vi "DataProcess_CalcTorque.vi"(8 "error in (no error)":errorcluster, 11 "Path":path) -> (0 "error out":errorcluster, 1 "AverageTorque":T1, 2 "Torques":T3, 3 "Torque Errors":T2, 5 "ExtraWeight(kg)":cluster{"Thigh":dbl, "Shank":dbl}, 7 "match substring":string)   [LabVIEW 2015]
uses:
  CAlex2-Data/CAlex2_Data.lvclass
  <vilib>/Analysis/5stat.llb/RMS (DBL).vi
  <vilib>/Analysis/NI_AALPro.lvlib
panel:
  out "Planned Torque 4":dbl[][](graph)
  out "Planned Torque 3":dbl[][](graph)
  out "PID Error":dbl[](array[numeric])
  out "Planning Error":dbl[](array[numeric])
  out "All Error":dbl[](array[numeric])
  out "Planed Torque":dbl[][](graph)
  out "Desired Torque":dbl[][](graph)
  out "Acutal Torque":dbl[][](graph)
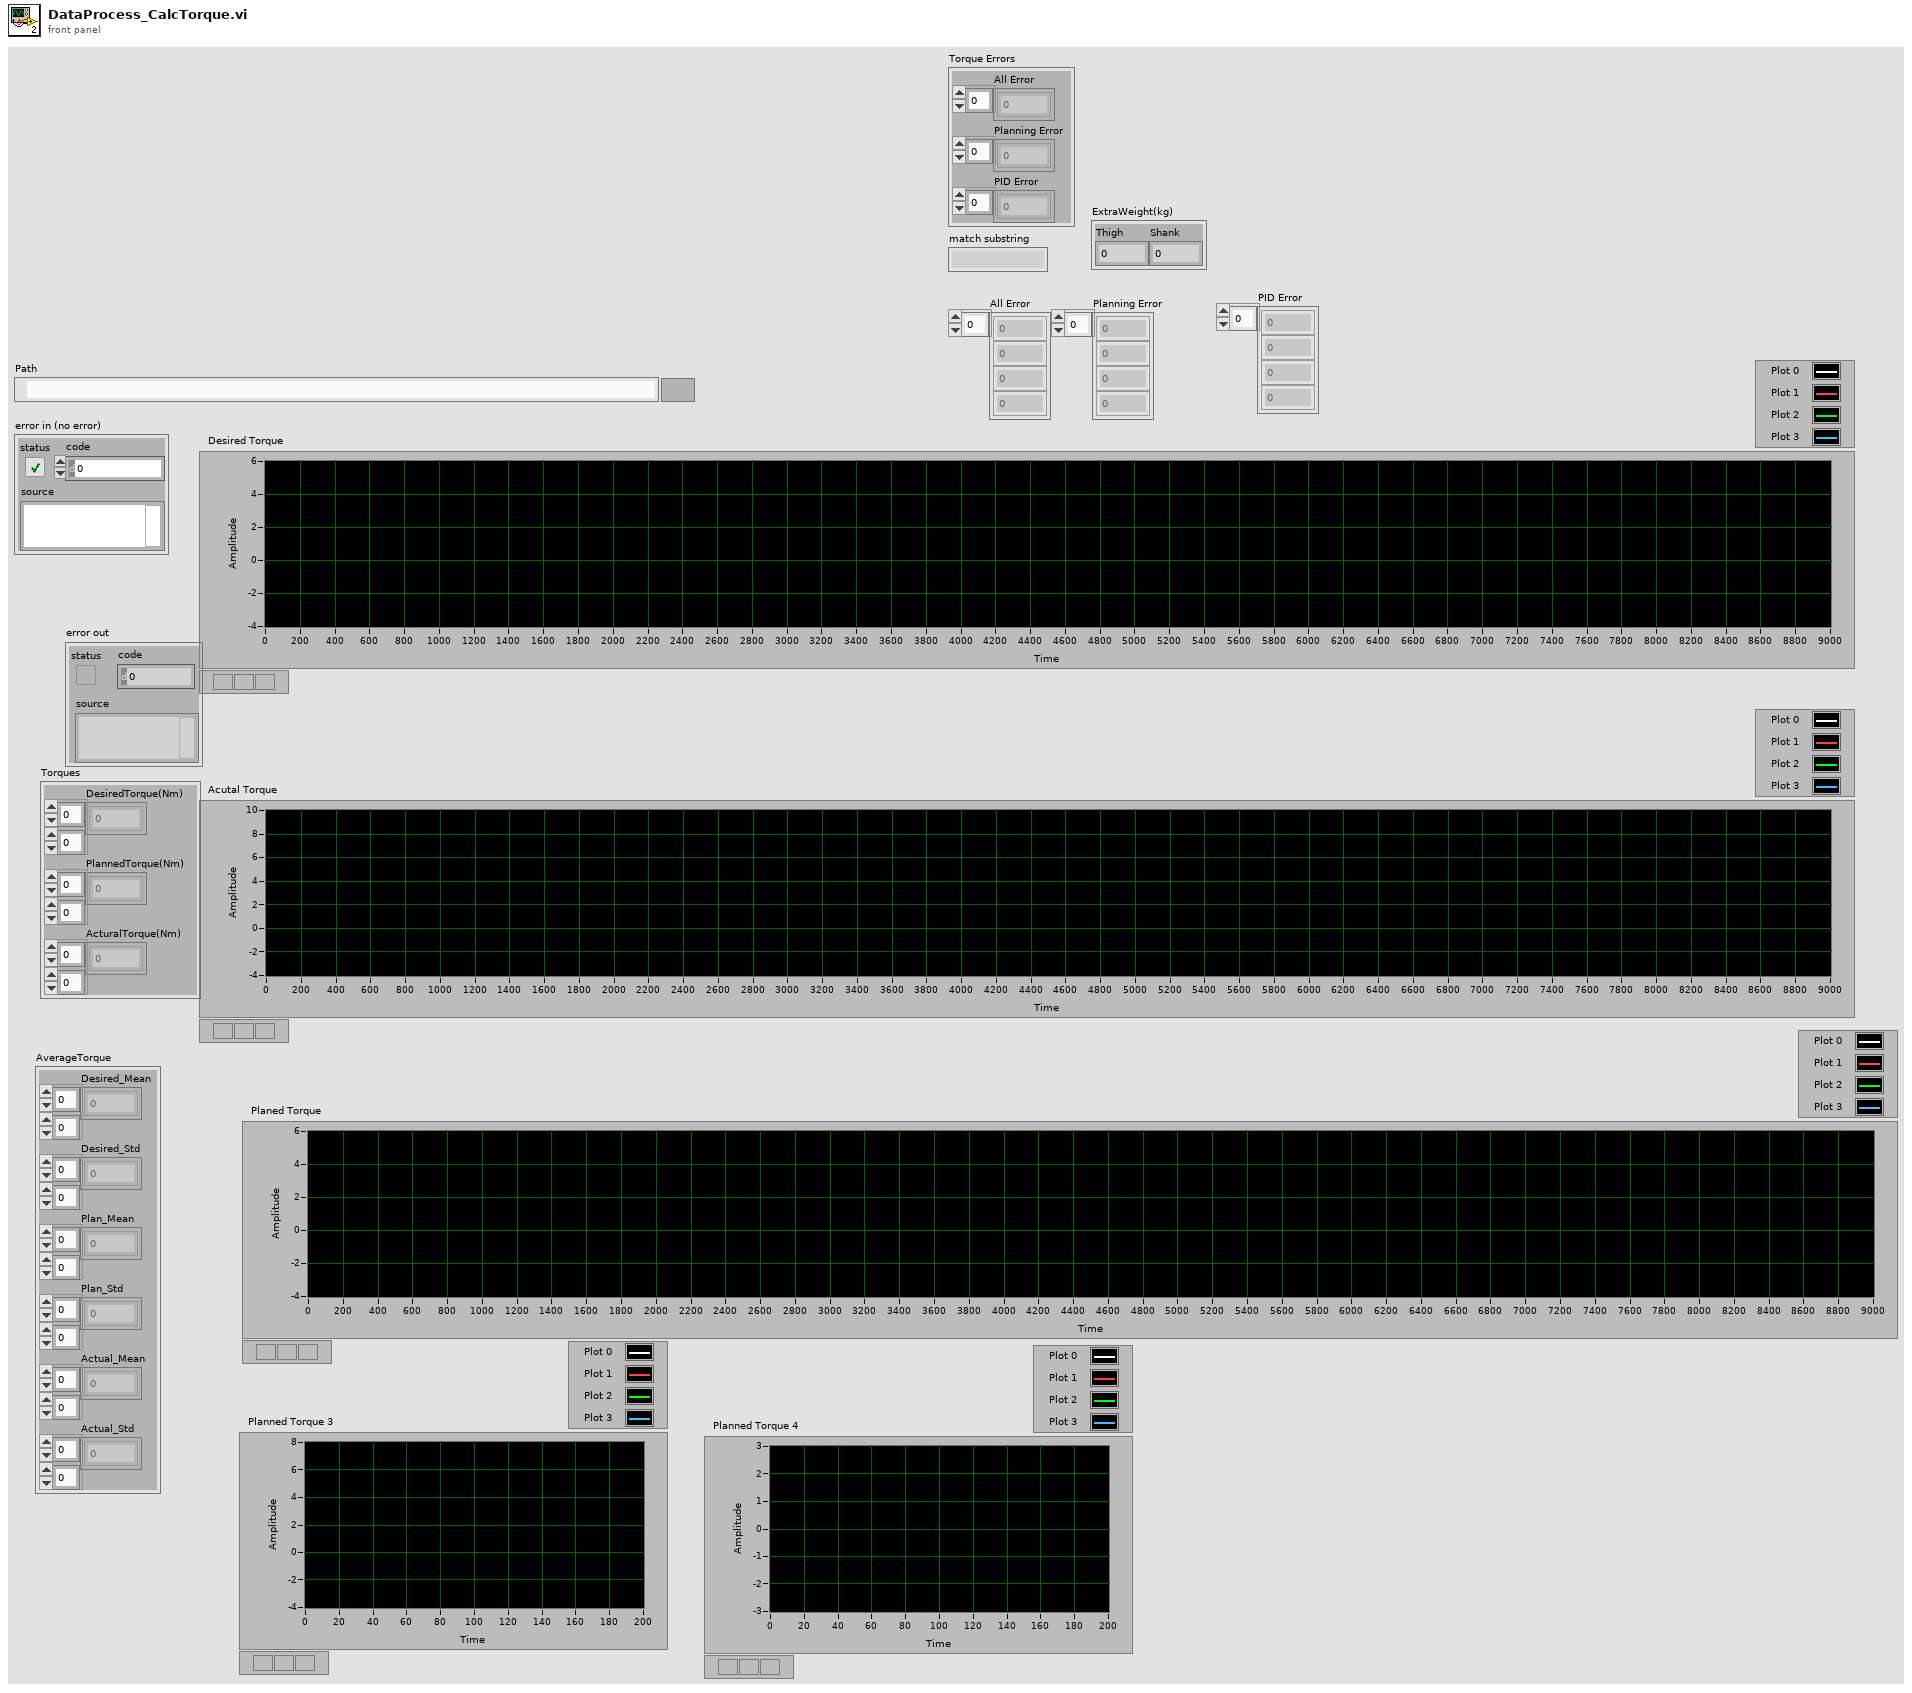
[diagram p1: front panel]
types:
  T1 = cluster{"Desired_Mean":dbl[][], "Desired_Std":dbl[][], "Plan_Mean":dbl[][], "Plan_Std":dbl[][], "Actual_Mean":dbl[][], "Actual_Std":dbl[][]}
  T2 = cluster{"All Error":dbl[], "Planning Error":dbl[], "PID Error":dbl[]}
  T3 = cluster{"DesiredTorque(Nm)":dbl[][], "PlannedTorque(Nm)":dbl[][], "ActuralTorque(Nm)":dbl[][]}
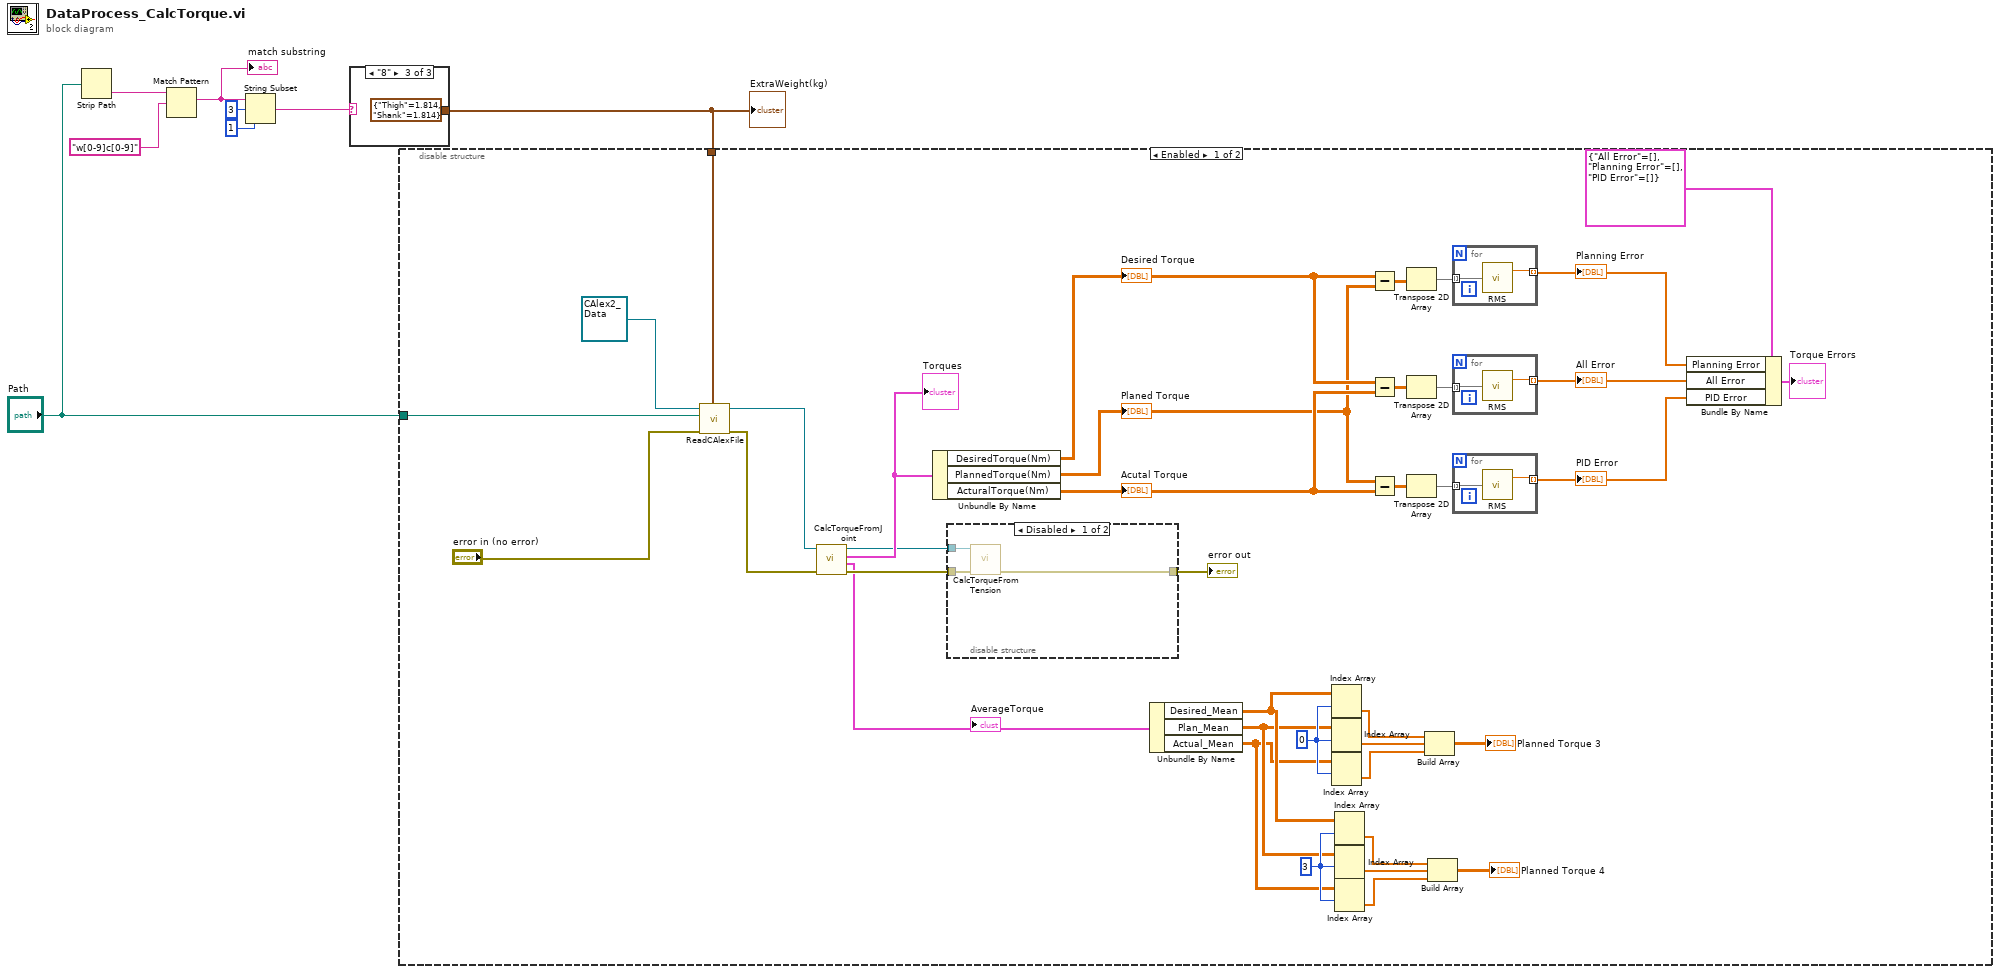
[diagram p0: block diagram]
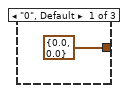
[diagram p4: hidden frame]
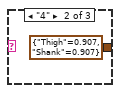
[diagram p5: hidden frame]
diagram:
  n1 = Strip Path(path="Path") -> (name=w7:string)  [unwired: 1 out]
  n2 = Match Pattern(string=w7, regular expression="w[0-9]c[0-9]") -> (match substring=w5:string)  [unwired: 1 in, 3 out]
  "match substring" <- w5
  n3 = String Subset(string=w5, offset (0)=3, length (rest)=1 ("length (rest)")) -> (substring=w2:string)
  n4 = case shown="\"8\"" w2 {
    tunnel: [cluster{"Thigh":dbl, "Shank":dbl} {"Thigh"=0.0, "Shank"=0.0} ("ExtraWeight(kg)") cluster{"Thigh":dbl, "Shank":dbl} {"Thigh"=0.907, "Shank"=0.907} ("ExtraWeight(kg)") cluster{"Thigh":dbl, "Shank":dbl} {"Thigh"=1.814, "Shank"=1.814} ("ExtraWeight(kg)")] -> w1
    frame "0", Default {
    }
    frame "4" {
    }
    frame "8" {
    }
  }
  "ExtraWeight(kg)" <- w1
  n5 = disable-structure shown="Enabled" {
    disable-tunnel: "Path" -> [w33 _]
    disable-tunnel: w1 -> [w31 _]
    frame Enabled {
      w19 = 3 ("index (row)")
      w20 = 0 ("index (row)")
      n6 = call "ReadCAlexFile.vi"("ExtraWeight(kg)"=w31, "error in (no error)"="error in (no error)", "ExpData File Path"=w33, "CAlexData2"=refnum<class "CAlex2_Data.lvclass"> refnum) -> ("error out"=w46:errorcluster, "CAlexData 2"=w47:refnum<class "CAlex2_Data.lvclass">)  [unwired: 6 in]
      n7 = call "CalcTorqueFromJoint.vi"("error in (no error)"=w46, "CAlexData2 in"=w47) -> ("error out"=w43:errorcluster, "AverageTorque"=w25:T1, "Torques"=w45:T3, "CarexMData out"=w44:refnum<class "CAlex2_Data.lvclass">)  [unwired: 5 in, 1 out]
      "Torques" <- w45
      "AverageTorque" <- w25
      n8 = Unbundle By Name(w45) -> ("DesiredTorque(Nm)"=w42:dbl[][], "PlannedTorque(Nm)"=w38:dbl[][], "ActuralTorque(Nm)"=w39:dbl[][])
      "Acutal Torque" <- w39
      "Desired Torque" <- w42
      "Planed Torque" <- w38
      n9 = disable-structure shown="Disabled" {
        disable-tunnel: w44 -> [w54 _]
        disable-tunnel: w43 -> [w53 w55]
        disable-tunnel: [w50 w55] -> w32
        frame Disabled {
          n10 = call "CalcTorqueFromTension.vi"("error in (no error)"=w53, "CAlexData2 in"=w54) -> ("error out"=w50:errorcluster, "Joint Torque Actual"=w51:dbl[][], "Joint Torque Desired"=w52:dbl[][])  [unwired: 4 in, 3 out]
        }
        frame Enabled {
        }
      }
      "error out" <- w32
      n11 = Unbundle By Name(w25) -> ("Desired_Mean"=w14:dbl[][], "Plan_Mean"=w13:dbl[][], "Actual_Mean"=w12:dbl[][])
      n12 = Index Array(array=w14, index (row)=w20) -> (element=w22:dbl[])  [unwired: 1 in]
      n13 = Index Array(array=w13, index (row)=w20) -> (element=w23:dbl[])  [unwired: 1 in]
      n14 = Index Array(array=w12, index (row)=w20) -> (element=w24:dbl[])  [unwired: 1 in]
      n15 = Index Array(array=w14, index (row)=w19) -> (element=w17:dbl[])  [unwired: 1 in]
      n16 = Index Array(array=w13, index (row)=w19) -> (element=w16:dbl[])  [unwired: 1 in]
      n17 = Index Array(array=w12, index (row)=w19) -> (element=w15:dbl[])  [unwired: 1 in]
      n18 = Subtract(x=w42, y=w38) -> (x-y=w41:dbl[][])
      n19 = Subtract(x=w42, y=w39) -> (x-y=w36:dbl[][])
      n20 = Subtract(x=w38, y=w39) -> (x-y=w34:dbl[][])
      n21 = Transpose 2D Array(2D array=w41) -> (transposed array=w40:dbl[][])
      n22 = Transpose 2D Array(2D array=w36) -> (transposed array=w37:dbl[][])
      n23 = Transpose 2D Array(2D array=w34) -> (transposed array=w35:dbl[][])
      n24 = Build Array(w22, w23, w24) -> (→"Planned Torque 3":dbl[][])
      n25 = Build Array(w17, w16, w15) -> (→"Planned Torque 4":dbl[][])
      n26 = for {
        tunnel: w40 -> [w61] mode=indexing
        tunnel: [w60] -> w30 mode=indexing
        n27 = call-poly <vilib>:"RMS.vi"("X"=w61) -> ("rms value"=w60:dbl)  [unwired: 1 out]
      }
      "Planning Error" <- w30
      n28 = for {
        tunnel: w37 -> [w59] mode=indexing
        tunnel: [w58] -> w29 mode=indexing
        n29 = call-poly <vilib>:"RMS.vi"("X"=w59) -> ("rms value"=w58:dbl)  [unwired: 1 out]
      }
      "All Error" <- w29
      n30 = for {
        tunnel: w35 -> [w57] mode=indexing
        tunnel: [w56] -> w28 mode=indexing
        n31 = call-poly <vilib>:"RMS.vi"("X"=w57) -> ("rms value"=w56:dbl)  [unwired: 1 out]
      }
      "PID Error" <- w28
      n32 = Bundle By Name(cluster=T2 {"All Error"=[], "Planning Error"=[], "PID Error"=[]}, "Planning Error"=w30, "All Error"=w29, "PID Error"=w28) -> (→"Torque Errors":T2)
    }
    frame Disabled {
    }
  }
